vi "Initialise.vi"(8 "error in (no error)":errorcluster, 10 "PC Messages Definitions File":path, 11 "PLC Messages Definitions File":path) -> (0 "error out":errorcluster, 3 "HMI Messages out":refnum<class "HMI Messages.lvclass">)   [LabVIEW 2015, in "HMI Messages.lvclass"]
uses:
  HMI Messages.lvclass
  HMI Messages.lvclass/HMI Messages.ctl
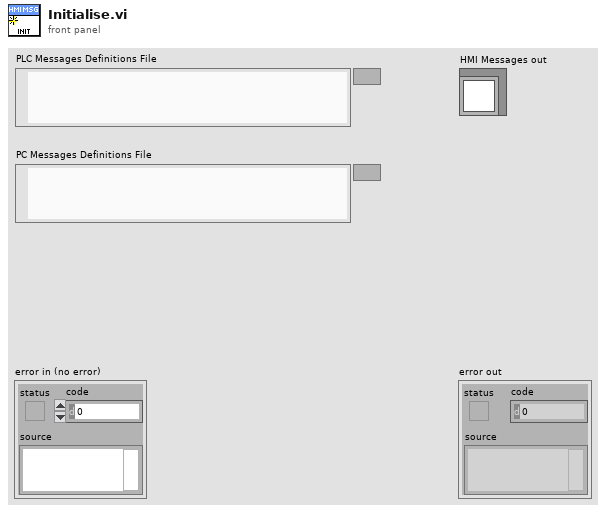
[diagram p1: front panel]
types:
  T1 = typedef "HMI Messages.lvclass/Message Definition.ctl" = cluster{"Number":i32, "Message":string}
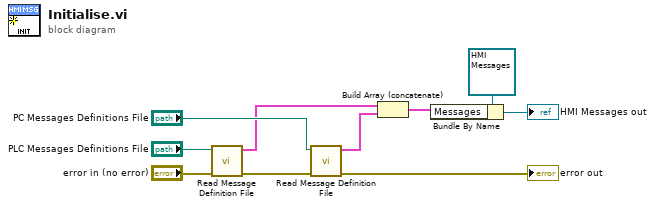
[diagram p0: block diagram]
diagram:
  n1 = call "Read Message Definition File.vi"("error in (no error)"="error in (no error)", "Messages Definitions File"="PLC Messages Definitions File") -> ("error out"=w9:errorcluster, "Messages"=w3:T1[])  [unwired: 8 in]
  n2 = call "Read Message Definition File.vi"("error in (no error)"=w9, "Messages Definitions File"="PC Messages Definitions File") -> ("error out"=→"error out":errorcluster, "Messages"=w2:T1[])  [unwired: 8 in]
  n3 = Build Array (concatenate)(w3, w2) -> (w1:T1[])
  n4 = Bundle By Name(cluster=refnum<class "HMI Messages.lvclass"> refnum ("HMI Messages out"), "Messages"=w1) -> (→"HMI Messages out":refnum<class "HMI Messages.lvclass">)
